vi "SelectConnections.vi"() -> (0 "Selected Connections":string[](array[string]))   [LabVIEW 2015]
panel:
  in  "EXIT":bool
  in  "RESET":bool
  in  "CONFIRM":bool
  out "Column":dbl=6.0
  out "Row":dbl=15.0
  in  "Devices":T1
  # "02"
  # "01"
  # "03"
  # "00"
  # "12"
  # "11"
  # "13"
  # "10"
  # "22"
  # "21"
  # "23"
  # "20"
  # "32"
  # "31"
  # "33"
  # "30"
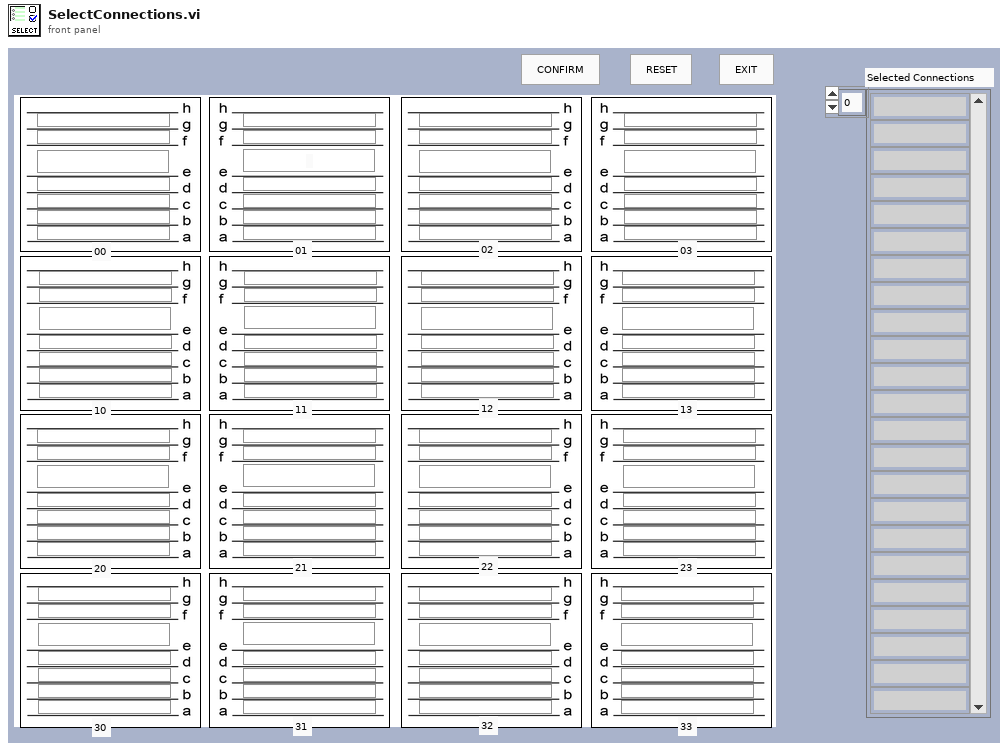
[diagram p1: front panel]
types:
  T1 = cluster{"00 Connections":cluster{"gh":bool, "fg":bool, "ef":bool, "de":bool, "cd":bool, "bc":bool, "ab":bool}, "01 Connections":cluster{"gh":bool, "fg":bool, "ef":bool, "de":bool, "cd":bool, "bc":bool, "ab":bool}, "02 Connections":cluster{"gh":bool, "fg":bool, "ef":bool, "de":bool, "cd":bool, "bc":bool, "ab":bool}, "03 Connections":cluster{"gh":bool, "fg":bool, "ef":bool, "de":bool, "cd":bool, "bc":bool, "ab":bool}, "10 Connections":cluster{"gh":bool, "fg":bool, "ef":bool, "de":bool, "cd":bool, "bc":bool, "ab":bool}, "11 Connections":cluster{"gh":bool, "fg":bool, "ef":bool, "de":bool, "cd":bool, "bc":bool, "ab":bool}, "12 Connections":cluster{"gh":bool, "fg":bool, "ef":bool, "de":bool, "cd":bool, "bc":bool, "ab":bool}, "13 Connections":cluster{"gh":bool, "fg":bool, "ef":bool, "de":bool, "cd":bool, "bc":bool, "ab":bool}, "20 Connections":cluster{"gh":bool, "fg":bool, "ef":bool, "de":bool, "cd":bool, "bc":bool, "ab":bool}, "21 Connections":cluster{"gh":bool, "fg":bool, "ef":bool, "de":bool, "cd":bool, "bc":bool, "ab":bool}, "22 Connections":cluster{"gh":bool, "fg":bool, "ef":bool, "de":bool, "cd":bool, "bc":bool, "ab":bool}, "23 Connections":cluster{"gh":bool, "fg":bool, "ef":bool, "de":bool, "cd":bool, "bc":bool, "ab":bool}, "30 Connections":cluster{"gh":bool, "fg":bool, "ef":bool, "de":bool, "cd":bool, "bc":bool, "ab":bool}, "31 Connections":cluster{"gh":bool, "fg":bool, "ef":bool, "de":bool, "cd":bool, "bc":bool, "ab":bool}, "32 Connections":cluster{"gh":bool, "fg":bool, "ef":bool, "de":bool, "cd":bool, "bc":bool, "ab":bool}, "33 Connections":cluster{"gh":bool, "fg":bool, "ef":bool, "de":bool, "cd":bool, "bc":bool, "ab":bool}}
  T2 = cluster{"gh":bool, "fg":bool, "ef":bool, "de":bool, "cd":bool, "bc":bool, "ab":bool}
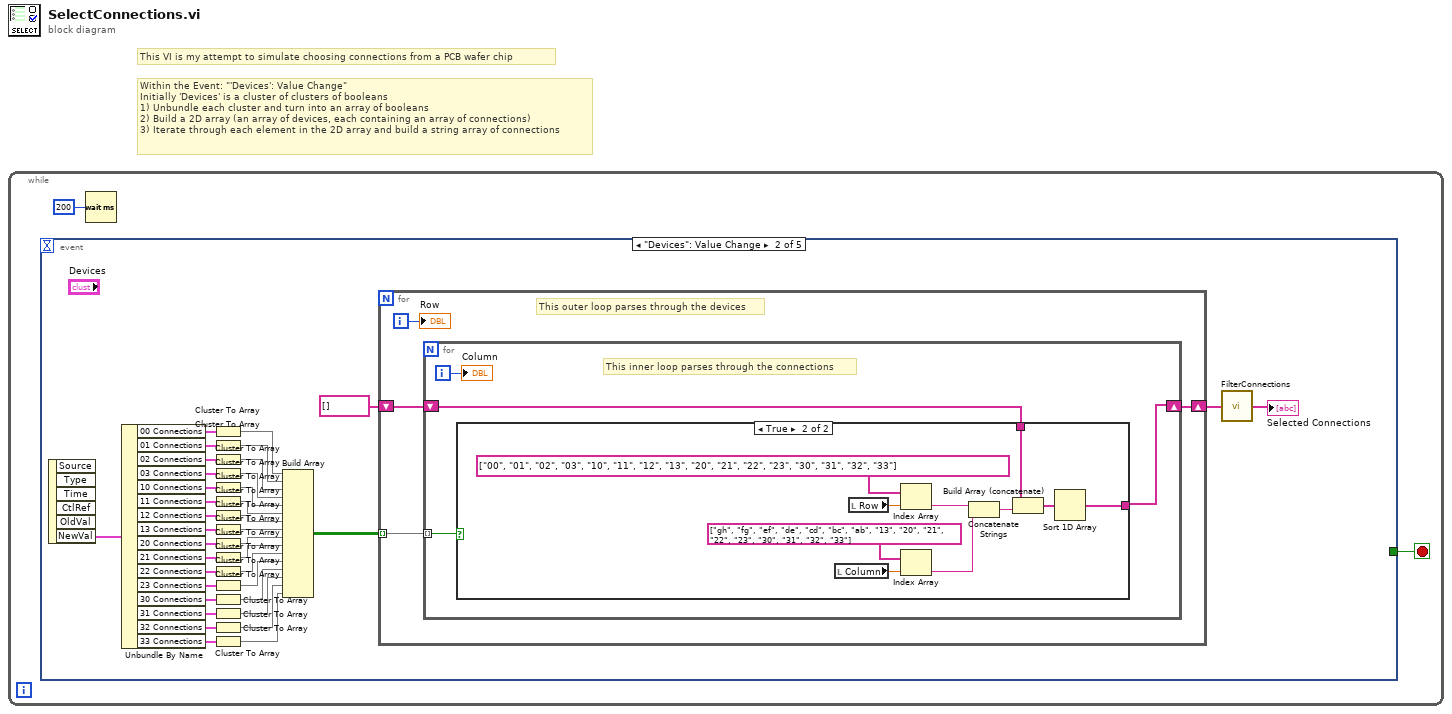
[diagram p0: block diagram]
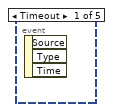
[diagram p2: hidden frame]
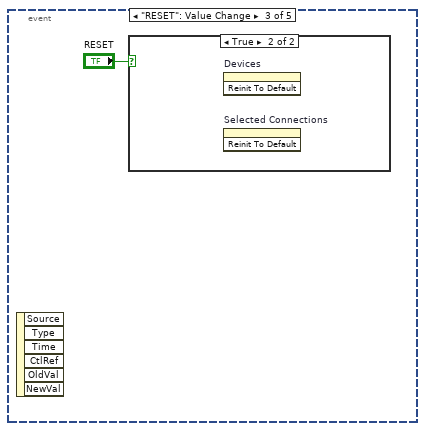
[diagram p4: hidden frame]
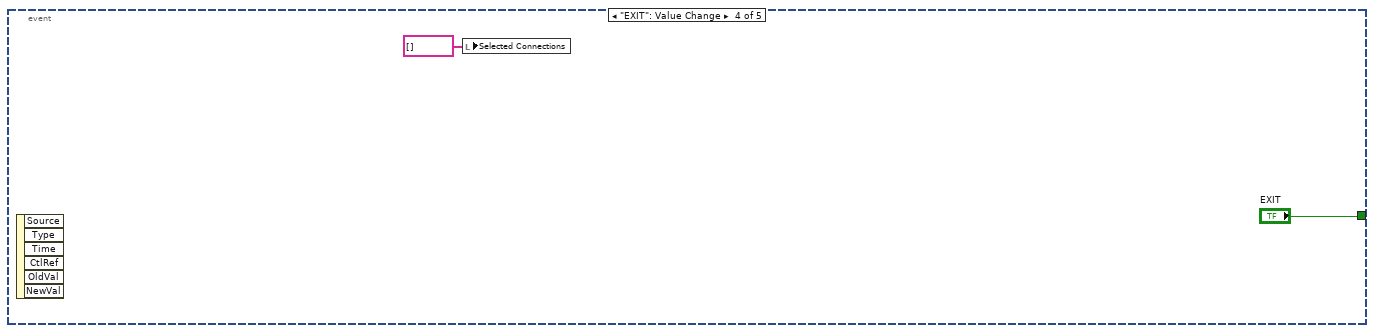
[diagram p6: hidden frame]
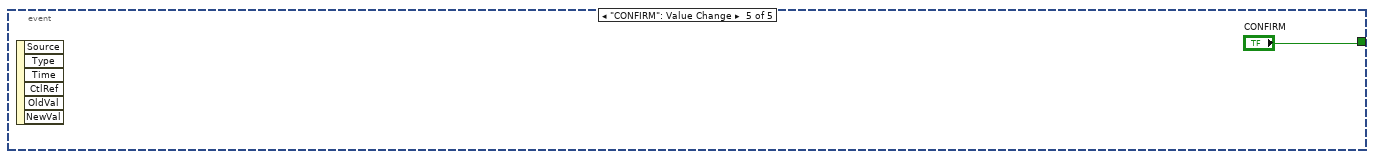
[diagram p7: hidden frame]
diagram:
  # "This VI is my attempt to simulate choosing connections from a PCB wafer chip"
  # "Within the Event: \"'Devices': Value Change\" \nInitially 'Devices' is a cluster of clusters of booleans\n1) Unbundle each cluster and turn into an array of booleans\n2) Build a 2D array (an array of devices, each containing an array of connections)\n3) Iterate through each element in the 2D array and build a string array of connections"
  n1 = while {
    stop <- w1 stop-if-true
    n2 = event shown="[1] \"Devices\": Value Change" {
      selector: _ -> [_ _ _ _ _]
      dyn-events: _ -> [_ _ _ _ _]
      timeout: _ -> [_ _ _ _ _]
      tunnel: [_ _ _ "EXIT" "CONFIRM"] -> w1
      event Timeout {
        n3 = event-data() -> ()  [unwired: 1 in, 3 out]
      }
      event "Devices": Value Change {
        n4 = event-data() -> ("NewVal"=w6:T1)  [unwired: 1 in, 5 out]
        n5 = Unbundle By Name(w6) -> ("00 Connections"=w39:T2, "01 Connections"=w38:T2, "02 Connections"=w37:T2, "03 Connections"=w36:T2, "10 Connections"=w35:T2, "11 Connections"=w34:T2, "12 Connections"=w33:T2, "13 Connections"=w32:T2, "20 Connections"=w31:T2, "21 Connections"=w30:T2, "22 Connections"=w29:T2, "23 Connections"=w28:T2, "30 Connections"=w27:T2, "31 Connections"=w26:T2, "32 Connections"=w25:T2, "33 Connections"=w24:T2)
        n6 = Cluster To Array(cluster=w39) -> (array=w23:bool[])
        n7 = Cluster To Array(cluster=w38) -> (array=w22:bool[])
        n8 = Cluster To Array(cluster=w37) -> (array=w21:bool[])
        n9 = Cluster To Array(cluster=w36) -> (array=w20:bool[])
        n10 = Cluster To Array(cluster=w35) -> (array=w19:bool[])
        n11 = Cluster To Array(cluster=w34) -> (array=w18:bool[])
        n12 = Cluster To Array(cluster=w33) -> (array=w17:bool[])
        n13 = Cluster To Array(cluster=w32) -> (array=w16:bool[])
        n14 = Cluster To Array(cluster=w31) -> (array=w15:bool[])
        n15 = Cluster To Array(cluster=w30) -> (array=w14:bool[])
        n16 = Cluster To Array(cluster=w29) -> (array=w13:bool[])
        n17 = Cluster To Array(cluster=w28) -> (array=w12:bool[])
        n18 = Cluster To Array(cluster=w27) -> (array=w11:bool[])
        n19 = Cluster To Array(cluster=w26) -> (array=w10:bool[])
        n20 = Cluster To Array(cluster=w25) -> (array=w9:bool[])
        n21 = Cluster To Array(cluster=w24) -> (array=w8:bool[])
        n22 = Build Array(w23, w22, w21, w20, w19, w18, w17, w16, w15, w14, w13, w12, w11, w10, w9, w8) -> (w7:bool[][])
        n23 = for {
          tunnel: w7 -> [w43] mode=indexing
          shift-right: [w41] -> w4
          shift-left: string[] [] -> [w40]
          i -> [w42]
          # "This outer loop parses through the devices"
          n24 = for {
            tunnel: w43 -> [w44] mode=indexing
            shift-right: [w46] -> w41
            shift-left: w40 -> [w45]
            i -> [w47]
            # "This inner loop parses through the connections"
            n25 = case shown="True" w44 {
              tunnel: [w48 w58] -> w46
              tunnel: w45 -> [w48 w57]
              frame False {
              }
              frame True {
                n26 = local read "Column"() -> (w55:dbl)
                n27 = local read "Row"() -> (w53:dbl)
                n28 = Index Array(array=string[] ["00", "01", "02", "03", "10", "11", "12", "13", "20", "21", "22", "23", "30", "31", "32", "33"], index=w53) -> (element=w50:string)
                n29 = Index Array(array=string[] ["gh", "fg", "ef", "de", "cd", "bc", "ab", "13", "20", "21", "22", "23", "30", "31", "32", "33"], index=w55) -> (element=w54:string)
                n30 = Concatenate Strings(w50, w54) -> (w51:string)
                n31 = Build Array (concatenate)(w57, w51) -> (w49:string[])
                n32 = Sort 1D Array(array=w49) -> (sorted array=w58:string[])
              }
            }
            "Column" <- w47
          }
          "Row" <- w42
        }
        n33 = call "FilterConnections.vi"("Selected Connections"=w4) -> ("Filtered Connections"=→"Selected Connections":string[])
      }
      event "RESET": Value Change {
        n34 = event-data() -> ()  [unwired: 1 in, 6 out]
        n35 = case shown="True" "RESET" {
          frame False {
          }
          frame True {
            n36 = invoke on="Devices" class="Clust (strict)" method="Reinit To Default"() -> ()  [unwired: 3 in, 3 out]
            n37 = invoke on="Selected Connections" class="Arr (strict)" method="Reinit To Default"() -> ()  [unwired: 3 in, 3 out]
          }
        }
      }
      event "EXIT": Value Change {
        n38 = event-data() -> ()  [unwired: 1 in, 6 out]
        n39 = local write "Selected Connections"(string[] [] ("Selected Connections")) -> ()
      }
      event "CONFIRM": Value Change {
        n40 = event-data() -> ()  [unwired: 1 in, 6 out]
      }
    }
    n41 = Wait (ms)(milliseconds to wait=u32 200) -> ()  [unwired: 1 out]
  }
